vi "StopVI.vi"(0 "vi reference in":refnum<vi>) -> (1 "responseXML":string="<?xml version=\"1.0\" encoding=\"UTF-8\"?>\n<methodResponse>\n\t<params>\n\t\t<param>\n\t\t\t<value><string>VI stopped</string></value>\n\t\t</param>\n\t</params>\n</methodResponse>\n", 2 "STATE":T1(ring))   [LabVIEW 2010]
panel:
  out "stopped?":bool
  out "error out":errorcluster
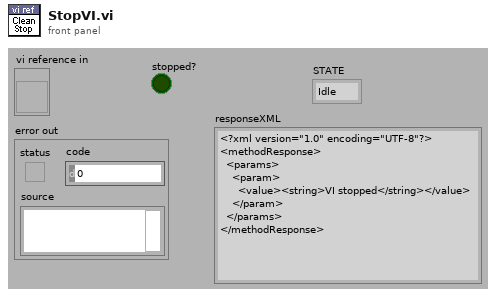
[diagram p1: front panel]
types:
  T1 = enum16{"Idle", "Connected", "Authenticated", "Opened", "Running", "Exit"}
  T2 = enum32{"Bad", "Idle", "Run top level", "Running"}
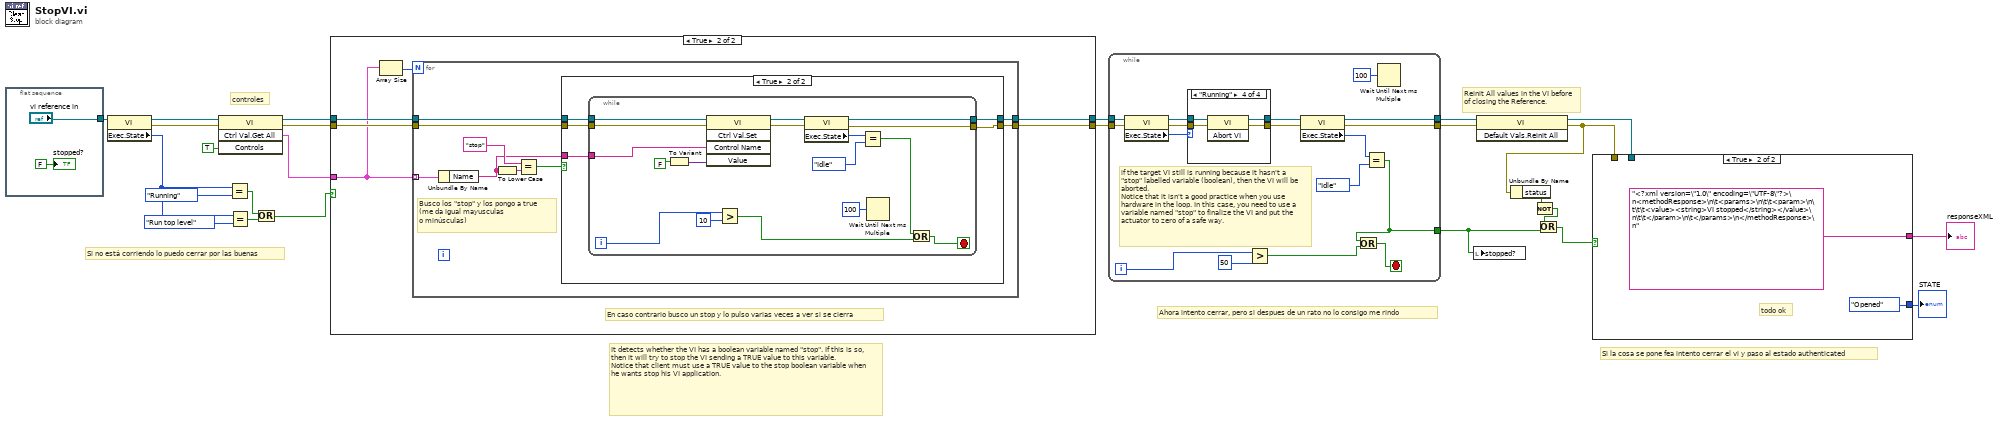
[diagram p0: block diagram]
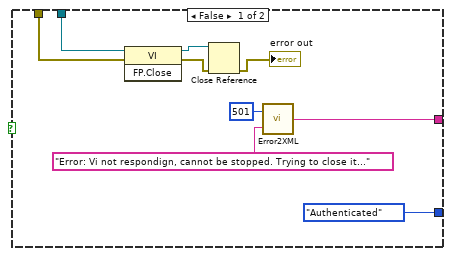
[diagram p2: hidden frame]
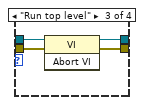
[diagram p5: hidden frame]
diagram:
  # "Si la cosa se pone fea intento cerrar el vi y paso al estado authenticated"
  # "Ahora intento cerrar, pero si despues de un rato no lo consigo me rindo"
  # "Si no está corriendo lo puedo cerrar por las buenas"
  # "controles"
  # "It detects whether the VI has a boolean variable named \"stop\". If this is so, then it will try to stop the VI sending a TRUE value to this variable.\nNotice that client must use a TRUE value to the stop boolean variable when he wants stop his VI application."
  # "Reinit All values in the VI before of closing the Reference."
  n1 = flat-sequence {
    tunnel: ["vi reference in"] -> w14
    frame #0 {
      "stopped?" <- FALSE ("stopped?")
    }
  }
  n2 = property class="VI"(reference=w14) -> (reference out=w13:refnum<vi>, error out=w12:errorcluster, "Exec.State"=w23:T2)  [unwired: 1 in]
  n3 = invoke class="VI" method="Ctrl Val.Get All"(reference=w13, error in=w12, "Controls"=TRUE) -> (reference out=w15:refnum<vi>, error out=w11:errorcluster, "Get All Control Values Variant"=w10:cluster{"Name":string, "Variant Data":variant}[])  [unwired: 1 in, 1 out]
  n4 = Equal?(x=w23, y=T2."Running") -> (x = y?=w24:bool)
  n5 = Equal?(x=w23, y=T2."Run top level") -> (x = y?=w21:bool)
  n6 = Or(x=w24, y=w21) -> (x .or. y?=w9:bool)
  n7 = case shown="True" w9 {
    tunnel: w10 -> [_ w30]
    tunnel: w15 -> [w29 w35]
    tunnel: w11 -> [w28 w34]
    tunnel: [w29 w33] -> w20
    tunnel: [w28 w32] -> w19
    frame False {
    }
    frame True {
      # "En caso contrario busco un stop y lo pulso varias veces a ver si se cierra"
      n8 = Array Size(array=w30) -> (size(s)=w31:i32)
      n9 = for {
        N: w31 -> [_]
        tunnel: w30 -> [w44] mode=indexing
        tunnel: w35 -> [w42]
        tunnel: w34 -> [w41]
        tunnel: [w39] -> w33
        tunnel: [w38] -> w32
        # "Busco los \"stop\" y los pongo a true\n(me da igual mayusculas\no minúsculas)"
        n10 = Unbundle By Name(w44) -> ("Name"=w36:string)
        n11 = To Lower Case(string=w36) -> (all lower case string=w37:string)
        n12 = Equal?(x="stop" ("y"), y=w37) -> (x = y?=w43:bool)
        n13 = case shown="True" w43 {
          tunnel: w42 -> [w46 w51]
          tunnel: w41 -> [w45 w50]
          tunnel: [w46 w49] -> w39
          tunnel: [w45 w48] -> w38
          tunnel: w36 -> [_ w47]
          frame False {
          }
          frame True {
            n14 = while {
              tunnel: w51 -> [w68]
              tunnel: w50 -> [w67]
              tunnel: [w61] -> w49
              tunnel: [w60] -> w48
              tunnel: w47 -> [w59]
              i -> [w54]
              stop <- w56 stop-if-true
              n15 = To Variant(anything=FALSE) -> (Variant=w58:variant)
              n16 = invoke class="VI" method="Ctrl Val.Set"(reference=w68, error in=w67, "Control Name"=w59, "Value"=w58) -> (reference out=w65:refnum<vi>, error out=w64:errorcluster)  [unwired: 1 in, 3 out]
              n17 = Greater?(x=w54, y=10) -> (0:w52:bool)
              n18 = property class="VI"(reference=w65, error in=w64) -> (reference out=w61:refnum<vi>, error out=w60:errorcluster, "Exec.State"=w63:T2)
              n19 = Equal?(x=w63, y=T2."Idle") -> (x = y?=w55:bool)
              n20 = Wait Until Next ms Multiple(millisecond multiple=u32 100) -> ()  [unwired: 1 out]
              n21 = Or(x=w55, y=w52) -> (x .or. y?=w56:bool)
            }
          }
        }
      }
    }
  }
  n22 = while {
    tunnel: w20 -> [w82]
    tunnel: w19 -> [w81]
    tunnel: [w78] -> w18
    tunnel: [w77] -> w17
    tunnel: [w69] -> w5
    i -> [w73]
    stop <- w71 stop-if-true
    # "if the target VI still is running because it hasn't a \"stop\" labelled variable (boolean), then the VI will be aborted.\nNotice that it isn't a good practice when you use hardware in the loop. In this case, you need to use a variable named \"stop\" to finalize the VI and put the actuator to zero of a safe way."
    n23 = property class="VI"(reference=w82, error in=w81) -> (reference out=w84:refnum<vi>, error out=w83:errorcluster, "Exec.State"=w85:T2)
    n24 = case shown="\"Running\"" w85 {
      tunnel: w84 -> [w87 w89 w93 w97]
      tunnel: w83 -> [w86 w88 w92 w96]
      tunnel: [w87 w89 w90 w95] -> w80
      tunnel: [w86 w88 w91 w94] -> w79
      frame "Bad", Default {
      }
      frame "Idle" {
      }
      frame "Run top level" {
        n25 = invoke class="VI" method="Abort VI"(reference=w93, error in=w92) -> (reference out=w90:refnum<vi>, error out=w91:errorcluster)  [unwired: 1 in, 1 out]
      }
      frame "Running" {
        n26 = invoke class="VI" method="Abort VI"(reference=w97, error in=w96) -> (reference out=w95:refnum<vi>, error out=w94:errorcluster)  [unwired: 1 in, 1 out]
      }
    }
    n27 = Greater?(x=w73, y=50) -> (0:w70:bool)
    n28 = property class="VI"(reference=w80, error in=w79) -> (reference out=w78:refnum<vi>, error out=w77:errorcluster, "Exec.State"=w75:T2)
    n29 = Equal?(x=w75, y=T2."Idle") -> (x = y?=w69:bool)
    n30 = Or(x=w69, y=w70) -> (x .or. y?=w71:bool)
    n31 = Wait Until Next ms Multiple(millisecond multiple=u32 100) -> ()  [unwired: 1 out]
  }
  n32 = local write "stopped?"(w5) -> ()
  n33 = invoke class="VI" method="Default Vals.Reinit All"(reference=w18, error in=w17) -> (reference out=w7:refnum<vi>, error out=w2:errorcluster)  [unwired: 1 in, 1 out]
  n34 = Unbundle By Name(w2) -> ("status"=w6:bool)
  n35 = Not(x=w6) -> (.not. x?=w4:bool)
  n36 = Or(x=w4, y=w5) -> (x .or. y?=w3:bool)
  n37 = case shown="True" w3 {
    tunnel: [w106 "<?xml version=\"1.0\" encoding=\"UTF-8\"?>\n<methodResponse>\n\t<params>\n\t\t<param>\n\t\t\t<value><string>VI stopped</string></value>\n\t\t</param>\n\t</params>\n</methodResponse>\n" ("ErrorXML")] -> w8
    tunnel: w7 -> [w103 _]
    tunnel: w2 -> [w102 _]
    tunnel: [T1."Authenticated" ("STATE") T1."Opened" ("STATE")] -> w1
    frame False {
      n38 = invoke class="VI" method="FP.Close"(reference=w103, error in=w102) -> (reference out=w101:refnum<vi>, error out=w100:errorcluster)  [unwired: 1 in, 1 out]
      n39 = Close Reference(reference=w101, error in (no error)=w100) -> (error out=→"error out":errorcluster)
      n40 = call "Error2XML.vi"("FailDescriptor"="Error: Vi not respondign, cannot be stopped. Trying to close it...", "FailID"=501) -> ("ErrorXML"=w106:string)
    }
    frame True {
      # "todo ok"
    }
  }
  "responseXML" <- w8
  "STATE" <- w1
